vi "Gen position coords array.vi"(8 "Error in":errorcluster, 10 "Number of rows to generate":i32=6, 11 "Experiment Parameters":T1={"Total Number of Miniscans"=1012, "Number of Trials"=20, "Number of cycles in a trial"=344, "Number of miniscans in a frame (Y)"=44, "Number of Pixels in Miniscan (X)"=85, "Number of Frames in Each Trial"=7912, "Number of Frames in a Cycle"=23, "DwellTime (us)"=0.05, "Acquisition length (sec)"=10.0}) -> (0 "error out":errorcluster, 3 "Coordinates of montage positions":cluster{"X\n\nY":i32[]}[](array[cluster]))   [LabVIEW 2017]
uses:
  Typedefs/Experiment Parameters.ctl
panel:
  out "Number of columns to generate":i32
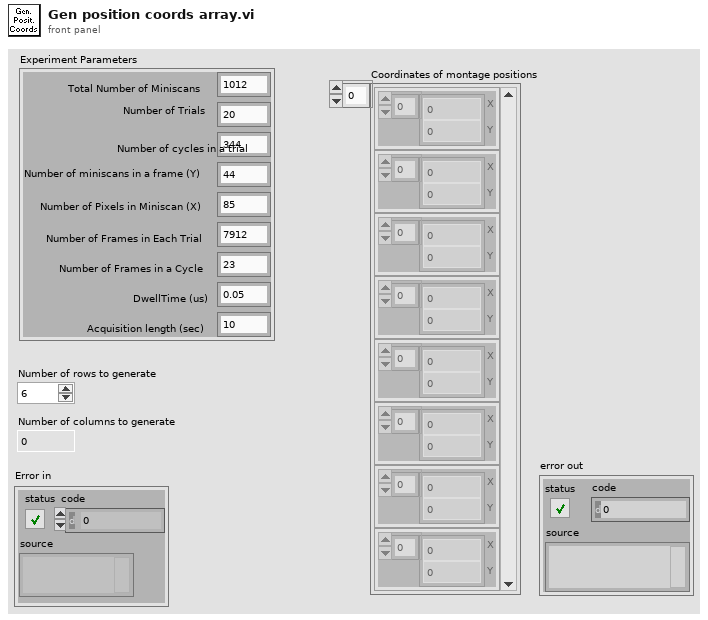
[diagram p1: front panel]
types:
  T1 = typedef "Experiment Parameters.ctl" = cluster{"Total Number of Miniscans":i32, "Number of Trials":i32, "Number of cycles in a trial":i32, "Number of miniscans in a frame (Y)":i32, "Number of Pixels in Miniscan (X)":i32, "Number of Frames in Each Trial":i32, "Number of Frames in a Cycle":i32, "DwellTime (us)":dbl, "Acquisition length (sec)":dbl}
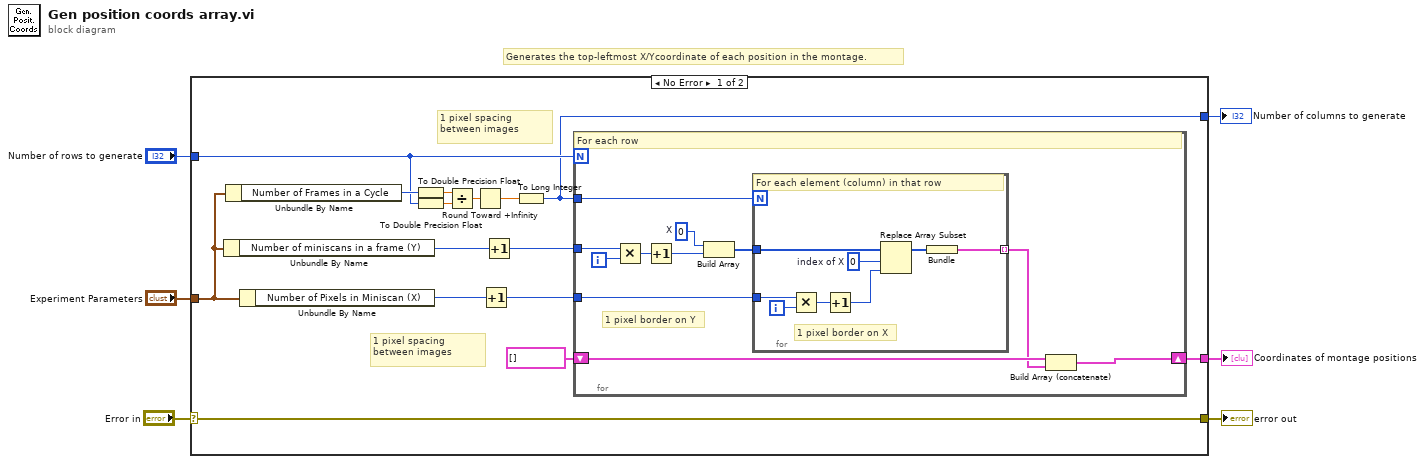
[diagram p0: block diagram]
diagram:
  # "Generates the top-leftmost X/Ycoordinate of each position in the montage."
  n1 = case shown="No Error" "Error in" {
    selector: "Error in" -> [w10 w41]
    tunnel: "Experiment Parameters" -> [w16 _]
    tunnel: "Number of rows to generate" -> [w15 _]
    tunnel: [w11 _] -> w4
    tunnel: [w10 w41] -> w2
    tunnel: [w9 _] -> w1
    frame No Error {
      # "1 pixel spacing between images"
      # "1 pixel spacing between images"
      n2 = Unbundle By Name(w16) -> ("Number of miniscans in a frame (Y)"=w14:i32)
      n3 = Unbundle By Name(w16) -> ("Number of Frames in a Cycle"=w20:i32)
      n4 = Unbundle By Name(w16) -> ("Number of Pixels in Miniscan (X)"=w13:i32)
      n5 = To Double Precision Float(number=w20) -> (double precision float=w18:dbl)
      n6 = To Double Precision Float(number=w15) -> (double precision float=w17:dbl)
      n7 = Divide(x=w18, y=w17) -> (x/y=w19:dbl)
      n8 = Round Toward +Infinity(x=w19) -> (ceil(x): smallest int >= x=w21:dbl)
      n9 = Increment(x=w13) -> (x+1=w7:i32)
      n10 = Increment(x=w14) -> (x+1=w8:i32)
      n11 = To Long Integer(number=w21) -> (32bit integer=w9:i32)
      n12 = for {
        N: w15 -> [_]
        tunnel: w9 -> [w32]
        tunnel: w8 -> [w29]
        tunnel: w7 -> [w26]
        shift-right: [w24] -> w11
        shift-left: cluster{"Offset Left/Top":i32[]}[] [] ("Coordinates of montage positions") -> [w25]
        i -> [w31]
        w27 = 0  # X
        # "1 pixel border on Y"
        # "For each row"
        n13 = Multiply(x=w29, y=w31) -> (x*y=w28:i32)
        n14 = Increment(x=w28) -> (x+1=w22:i32)
        n15 = Build Array(w27, w22) -> (w30:i32[])
        n16 = for {
          N: w32 -> [_]
          tunnel: w30 -> [w40]
          tunnel: w26 -> [w37]
          tunnel: [w34] -> w23 mode=indexing
          i -> [w38]
          w39 = 0  # index of X
          # "1 pixel border on X"
          # "For each element (column) in that row"
          n17 = Multiply(x=w37, y=w38) -> (x*y=w36:i32)
          n18 = Increment(x=w36) -> (x+1=w33:i32)
          n19 = Replace Array Subset "Replace Array Subset"(array=w40, new element=w33, index=w39) -> (w35:i32[])
          n20 = Bundle(w35) -> (w34:cluster{i32[]})  [unwired: 1 in]
        }
        n21 = Build Array (concatenate)(w25, w23) -> (w24:cluster{"Offset Left/Top":i32[]}[])
      }
    }
    frame Error {
    }
  }
  "Coordinates of montage positions" <- w4
  "error out" <- w2
  "Number of columns to generate" <- w1
